vi "initialize hardware.vi"(7 "Reset (False)":bool, 8 "error in (no error)":errorcluster, 9 "devport":string, 10 "Settings":T1={"devport"="", "Position"={"Axis 1"={"Value"=0.0, "Min"=0.0, "Max"=0.0, "StepSize"=0.0, "Tolerance"=0.0, "ValueActual"=0.0}, "Axis 2"={"Value"=0.0, "Min"=0.0, "Max"=0.0, "StepSize"=0.0, "Tolerance"=0.0, "ValueActual"=0.0}, "Axis 3"={"Value"=0.0, "Min"=0.0, "Max"=0.0, "StepSize"=0.0, "Tolerance"=0.0, "ValueActual"=0.0}}, "Power"={"Axis 1"=enum."off", "Axis 2"=enum."off", "Axis 3"=enum."off"}, "Status"={"Axis 1"=enum."Not referenced", "Axis 2"=enum."Not referenced", "Axis 3"=enum."Not referenced"}, "Backlash"={"Axis 1"={"Value"=0.0, "Min"=0.0, "Max"=0.0, "StepSize"=0.0, "Tolerance"=0.0, "ValueActual"=0.0}, "Axis 2"={"Value"=0.0, "Min"=0.0, "Max"=0.0, "StepSize"=0.0, "Tolerance"=0.0, "ValueActual"=0.0}, "Axis 3"={"Value"=0.0, "Min"=0.0, "Max"=0.0, "StepSize"=0.0, "Tolerance"=0.0, "ValueActual"=0.0}}, "Home"={"Axis 1"={"Value"=0.0, "Min"=0.0, "Max"=0.0, "StepSize"=0.0, "Tolerance"=0.0, "ValueActual"=0.0}, "Axis 2"={"Value"=0.0, "Min"=0.0, "Max"=0.0, "StepSize"=0.0, "Tolerance"=0.0, "ValueActual"=0.0}, "Axis 3"={"Value"=0.0, "Min"=0.0, "Max"=0.0, "StepSize"=0.0, "Tolerance"=0.0, "ValueActual"=0.0}}, "MoveToHardLimit"={"Axis 1"=enum."pos", "Axis 2"=enum."pos", "Axis 3"=enum."pos"}, "relativeMove"={"Axis 1neg"=enum."off", "Axis 2neg"=enum."off", "Axis 3neg"=enum."off", "Axis 1pos"=enum."off", "Axis 2pos"=enum."off", "Axis 3pos"=enum."off"}, "stepsize"={"Value"=0.0, "Min"=0.0, "Max"=0.0, "StepSize"=0.0, "Tolerance"=0.0, "ValueActual"=0.0}, "automotoroff"=enum."off", "ResetBeforeMove"=enum."off", "Enable"={"Axis 1"=enum."on", "Axis 2"=enum."on", "Axis 3"=enum."on"}}, 11 "ESP301 in":refnum<class "ESP301.lvclass">) -> (0 "error out":errorcluster, 2 "VISA resource name out":refnum<visa-resource-name>, 3 "ESP301 out":refnum<class "ESP301.lvclass">)   [LabVIEW 2020, in "ESP301.lvclass"]
uses:
  ESP301.lvclass
  SettingsTypdef.ctl
  shared/OnOffTypeDef.ctl
  status_TypDef.ctl
  Hardware limit.ctl
  ESP301.lvclass/ESP301.ctl
  shared/CompressAndUpdate(Poly)/CompressAndUpdate(Enum).vi
  shared/CompressAndUpdate(Poly)/CompressAndUpdate(Numeric).vi
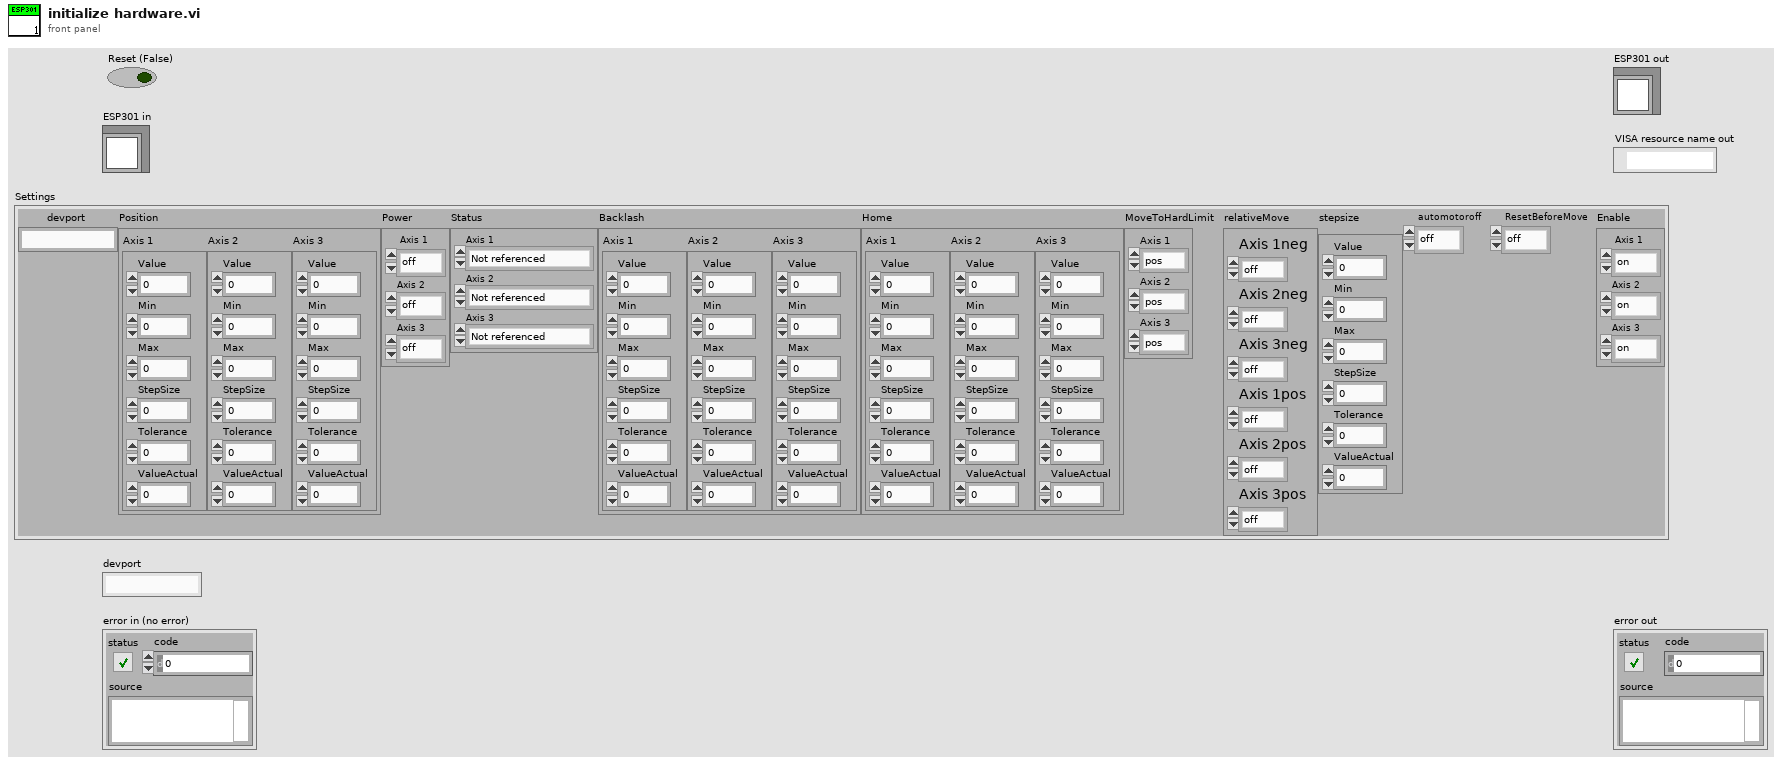
[diagram p1: front panel]
types:
  T1 = typedef "ESP301.lvclass/SettingsTypdef.ctl" = cluster{"devport":string, "Position":cluster{"Axis 1":cluster{"Value":dbl, "Min":dbl, "Max":dbl, "StepSize":dbl, "Tolerance":dbl, "ValueActual":dbl}, "Axis 2":cluster{"Value":dbl, "Min":dbl, "Max":dbl, "StepSize":dbl, "Tolerance":dbl, "ValueActual":dbl}, "Axis 3":cluster{"Value":dbl, "Min":dbl, "Max":dbl, "StepSize":dbl, "Tolerance":dbl, "ValueActual":dbl}}, "Power":cluster{"Axis 1":T2, "Axis 2":T2, "Axis 3":T2}, "Status":cluster{"Axis 1":T3, "Axis 2":T3, "Axis 3":T3}, "Backlash":cluster{"Axis 1":cluster{"Value":dbl, "Min":dbl, "Max":dbl, "StepSize":dbl, "Tolerance":dbl, "ValueActual":dbl}, "Axis 2":cluster{"Value":dbl, "Min":dbl, "Max":dbl, "StepSize":dbl, "Tolerance":dbl, "ValueActual":dbl}, "Axis 3":cluster{"Value":dbl, "Min":dbl, "Max":dbl, "StepSize":dbl, "Tolerance":dbl, "ValueActual":dbl}}, "Home":cluster{"Axis 1":cluster{"Value":dbl, "Min":dbl, "Max":dbl, "StepSize":dbl, "Tolerance":dbl, "ValueActual":dbl}, "Axis 2":cluster{"Value":dbl, "Min":dbl, "Max":dbl, "StepSize":dbl, "Tolerance":dbl, "ValueActual":dbl}, "Axis 3":cluster{"Value":dbl, "Min":dbl, "Max":dbl, "StepSize":dbl, "Tolerance":dbl, "ValueActual":dbl}}, "MoveToHardLimit":cluster{"Axis 1":T4, "Axis 2":T4, "Axis 3":T4}, "relativeMove":cluster{"Axis 1neg":T2, "Axis 2neg":T2, "Axis 3neg":T2, "Axis 1pos":T2, "Axis 2pos":T2, "Axis 3pos":T2}, "stepsize":cluster{"Value":dbl, "Min":dbl, "Max":dbl, "StepSize":dbl, "Tolerance":dbl, "ValueActual":dbl}, "automotoroff":T2, "ResetBeforeMove":T2, "Enable":cluster{"Axis 1":T2, "Axis 2":T2, "Axis 3":T2}}
  T2 = typedef "OnOffTypeDef.ctl" = enum16{"off", "on"}
  T3 = typedef "status_TypDef.ctl" = enum16{"Not referenced", "Homing", "Moving", "Ready"}
  T4 = typedef "Hardware limit.ctl" = enum16{"pos", "neg"}
  T5 = cluster{"Axis 1":cluster{"Value":dbl, "Min":dbl, "Max":dbl, "StepSize":dbl, "Tolerance":dbl, "ValueActual":dbl}, "Axis 2":cluster{"Value":dbl, "Min":dbl, "Max":dbl, "StepSize":dbl, "Tolerance":dbl, "ValueActual":dbl}, "Axis 3":cluster{"Value":dbl, "Min":dbl, "Max":dbl, "StepSize":dbl, "Tolerance":dbl, "ValueActual":dbl}}
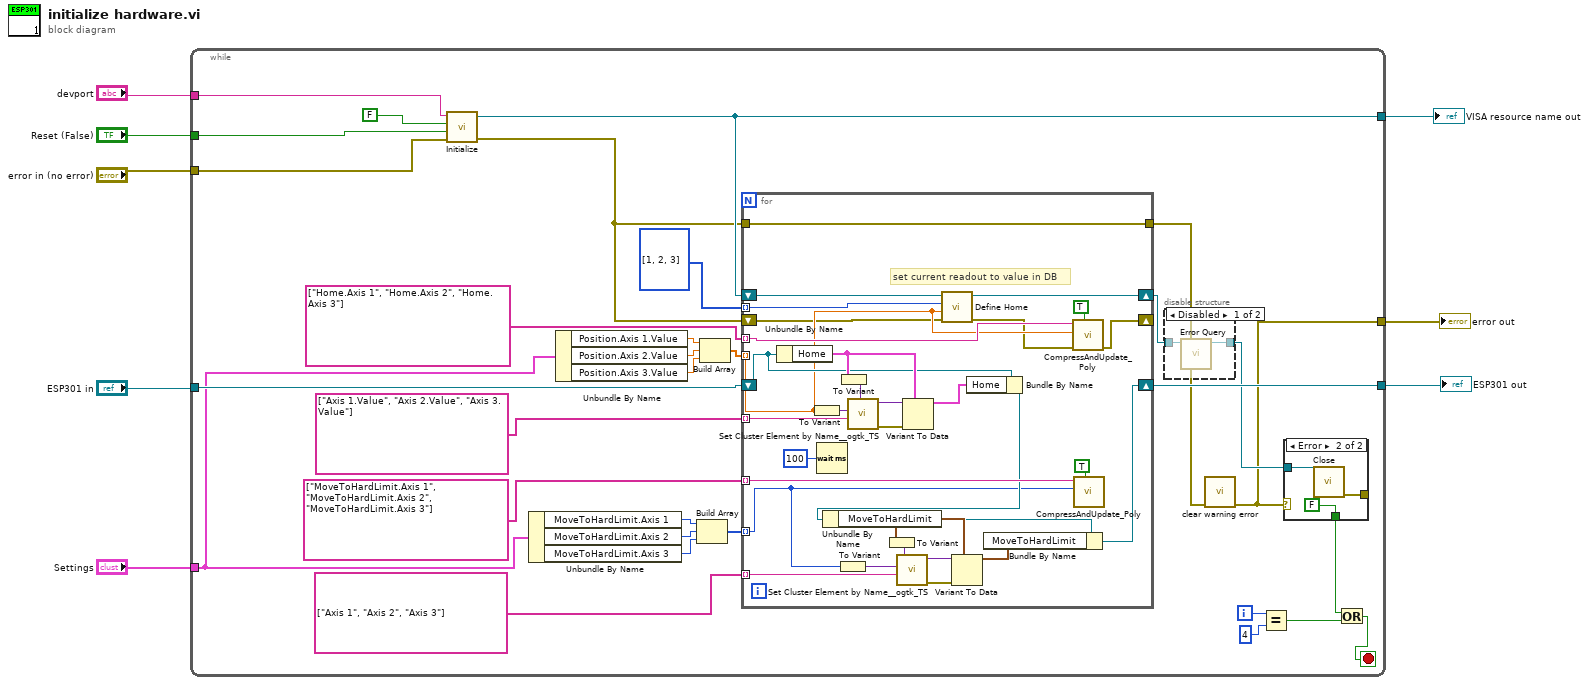
[diagram p0: block diagram]
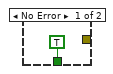
[diagram p3: hidden frame]
diagram:
  n1 = while {
    tunnel: "error in (no error)" -> [w11]
    tunnel: "devport" -> [w14]
    tunnel: "ESP301 in" -> [w34]
    tunnel: [w33] -> w4
    tunnel: [w13] -> w5
    tunnel: "Settings" -> [w23]
    tunnel: [w17] -> w7
    tunnel: "Reset (False)" -> [w9]
    i -> [w22]
    stop <- w19 stop-if-true
    n2 = call "Initialize.vi"("VISA resource name"=w14, "ID Query (True)"=FALSE, "Reset (False)"=w9, "error in (no error)"=w11) -> ("VISA resource name out"=w13:refnum<visa-resource-name>, "error out"=w12:errorcluster)  [unwired: 5 in]
    n3 = Unbundle By Name(w23) -> ("MoveToHardLimit.Axis 1"=w26:T4, "MoveToHardLimit.Axis 2"=w27:T4, "MoveToHardLimit.Axis 3"=w28:T4)
    n4 = Unbundle By Name(w23) -> ("Position.Axis 1.Value"=w38:dbl, "Position.Axis 2.Value"=w37:dbl, "Position.Axis 3.Value"=w36:dbl)
    n5 = Build Array(w26, w27, w28) -> (w25:T4[])
    n6 = Build Array(w38, w37, w36) -> (w35:dbl[])
    n7 = for {
      shift-right: [w68] -> w30
      shift-left: w13 -> [w69]
      tunnel: i32[] [1, 2, 3] -> [w67] mode=indexing
      tunnel: w35 -> [w66] mode=indexing
      shift-right: [w55] -> w33
      shift-left: w34 -> [w73]
      tunnel: string[] ["Axis 1.Value", "Axis 2.Value", "Axis 3.Value"] ("set following Variables (empty = all avriables)") -> [w72] mode=indexing
      tunnel: string[] ["Home.Axis 1", "Home.Axis 2", "Home.Axis 3"] ("set following Variables (empty = all avriables)") -> [w70] mode=indexing
      shift-right: [w63] -> _
      shift-left: w12 -> [w65]
      tunnel: string[] ["MoveToHardLimit.Axis 1", "MoveToHardLimit.Axis 2", "MoveToHardLimit.Axis 3"] ("set following Variables (empty = all avriables)") -> [w61] mode=indexing
      tunnel: w25 -> [w54] mode=indexing
      tunnel: string[] ["Axis 1", "Axis 2", "Axis 3"] ("set following Variables (empty = all avriables)") -> [w53] mode=indexing
      tunnel: w12 -> [w51]
      tunnel: [w51] -> w15
      # "set current readout to value in DB"
      n8 = Unbundle By Name(w73) -> ("Home"=w76:T5)
      n9 = To Variant(anything=w66) -> (Variant=w48:variant)
      n10 = Wait (ms)(milliseconds to wait=u32 100) -> ()  [unwired: 1 out]
      n11 = To Variant(anything=w54) -> (Variant=w49:variant)
      n12 = To Variant(anything=w76) -> (Variant=w47:variant)
      n13 = call "Set Cluster Element by Name__ogtk_TS.vi"("Element Name (\"\": New Element Data Name)"=w72, "New Element Value"=w48, "Cluster"=w47) -> ("error out"=w74:errorcluster, "VCluster out"=w75:variant)  [unwired: 6 in, 1 out]
      n14 = Variant To Data(error in=w74, type=w76, Variant=w75) -> (data=w77:T5)  [unwired: 1 out]
      n15 = call "Define Home.vi"("error in (no error)"=w65, "Home Position (0 units)"=w66, "Axis (1)"=w67, "VISA resource name"=w69) -> ("error out"=w64:errorcluster, "VISA resource name out"=w68:refnum<visa-resource-name>)  [unwired: 2 in]
      n16 = Bundle By Name(cluster=w73, "Home"=w77) -> (w56:refnum<class "ESP301.lvclass">)
      n17 = Unbundle By Name(w56) -> ("MoveToHardLimit"=w58:cluster{"Axis 1":T4, "Axis 2":T4, "Axis 3":T4})
      n18 = To Variant(anything=w58) -> (Variant=w50:variant)
      n19 = call "Set Cluster Element by Name__ogtk_TS.vi"("Element Name (\"\": New Element Data Name)"=w53, "New Element Value"=w49, "Cluster"=w50) -> ("error out"=w60:errorcluster, "VCluster out"=w59:variant)  [unwired: 6 in, 1 out]
      n20 = Variant To Data(error in=w60, type=w58, Variant=w59) -> (data=w57:cluster{"Axis 1":T4, "Axis 2":T4, "Axis 3":T4})  [unwired: 1 out]
      n21 = Bundle By Name(cluster=w56, "MoveToHardLimit"=w57) -> (w55:refnum<class "ESP301.lvclass">)
      n22 = call-poly "CompressAndUpdate_Poly.vi"("force CVT update (false)"=TRUE ("force CVT update"), "error in"=w64, "Numeric"=w66, "command or variable name"=w70) -> ("error out"=w63:errorcluster)  [unwired: 7 in]
      n23 = call-poly "CompressAndUpdate_Poly.vi"("force CVT update (false)"=TRUE ("force CVT update"), "enum variant"=w54, "command or variable name"=w61) -> ()  [unwired: 8 in, 1 out]
    }
    n24 = disable-structure shown="Disabled" {
      disable-tunnel: w30 -> [w41 w42]
      disable-tunnel: [w40 w42] -> w18
      frame Disabled {
        n25 = call "Error Query.vi"("VISA resource name"=w41) -> ("VISA resource name out"=w40:refnum<visa-resource-name>)  [unwired: 3 in, 3 out]
      }
      frame Enabled {
      }
    }
    n26 = call "clear warning error.vi"("error in"=w15) -> ("error out"=w17:errorcluster)  [unwired: 10 in]
    n27 = Equal?(x=w22, y=4) -> (x = y?=w20:bool)
    n28 = case shown="Error" w17 {
      tunnel: w18 -> [_ w45]
      tunnel: [TRUE FALSE] -> w16
      tunnel: [_ w44] -> _
      frame No Error {
      }
      frame Error {
        n29 = call "Close.vi"("VISA resource name"=w45) -> ("error out"=w44:errorcluster)  [unwired: 10 in]
      }
    }
    n30 = Or(x=w16, y=w20) -> (x .or. y?=w19:bool)
  }
  "error out" <- w7
  "VISA resource name out" <- w5
  "ESP301 out" <- w4
